vi "FormMain.vi"() -> ()   [LabVIEW 2013]
uses:
  resultShow.vi
panel:
  in  "FormProductsTable":bool
  in  "B030管理":bool
  out "rigStatus 2":string="提示信息"
  in  "判定设定 2":string[][](table)
  in  "参数设定 2":string[][](table)
  out "takesTime":string
  out "表格控件":string[][](table)
  out "FFT范围 2":string[][](table)
  out "输出扭矩":dbl caption="数值 24" format="%.1f Nm"
  in  "打开按钮":bool
  out "rigStatus":string="提示信息"
  out "connectionMode":string
  out "productsName":string
  out "userStatus":string
  out "userName":string
  # "电机/控制器专配专机"
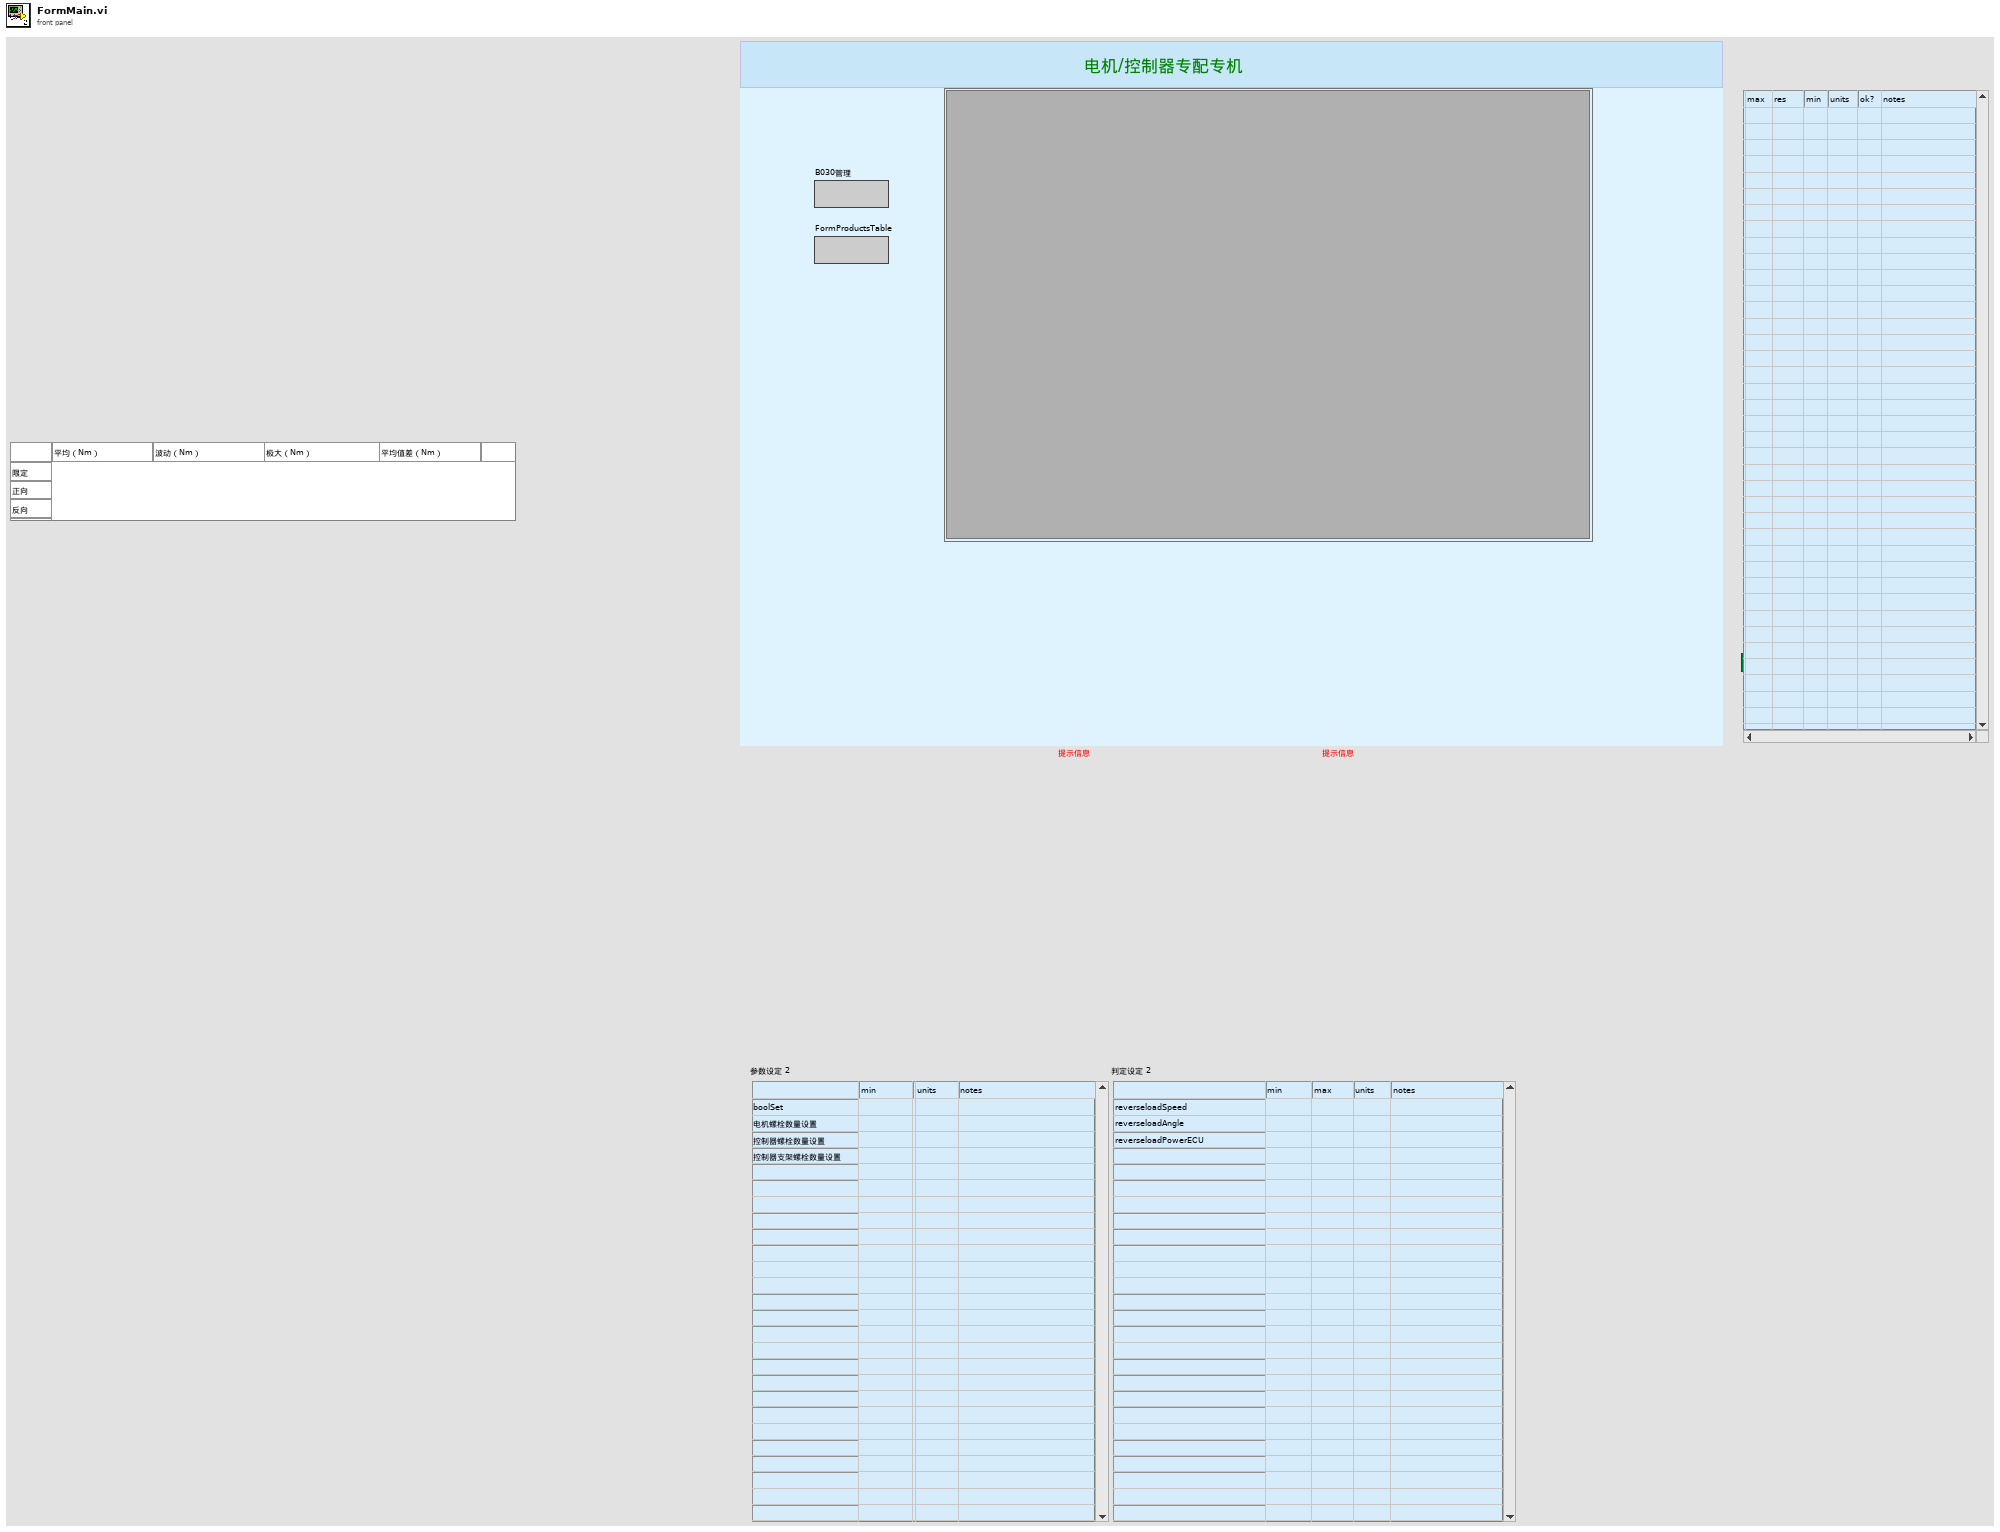
[diagram p1: front panel]
types:
  T1 = enum32{"Invalid", "Standard", "Closed", "Hidden", "Minimized", "Maximized"}
  T2 = cluster{"userCode":string, "userName":string, "userStatus":string, "connectionMode":string, "takesTime":string, "countDone":string, "countOK":string, "countNG":string, "rigStatus":string, "productsName":string, "partCode1":string, "partCode2":string, "partCode3":string}
  T3 = enum32{"Bad", "Idle", "Run top level", "Running"}
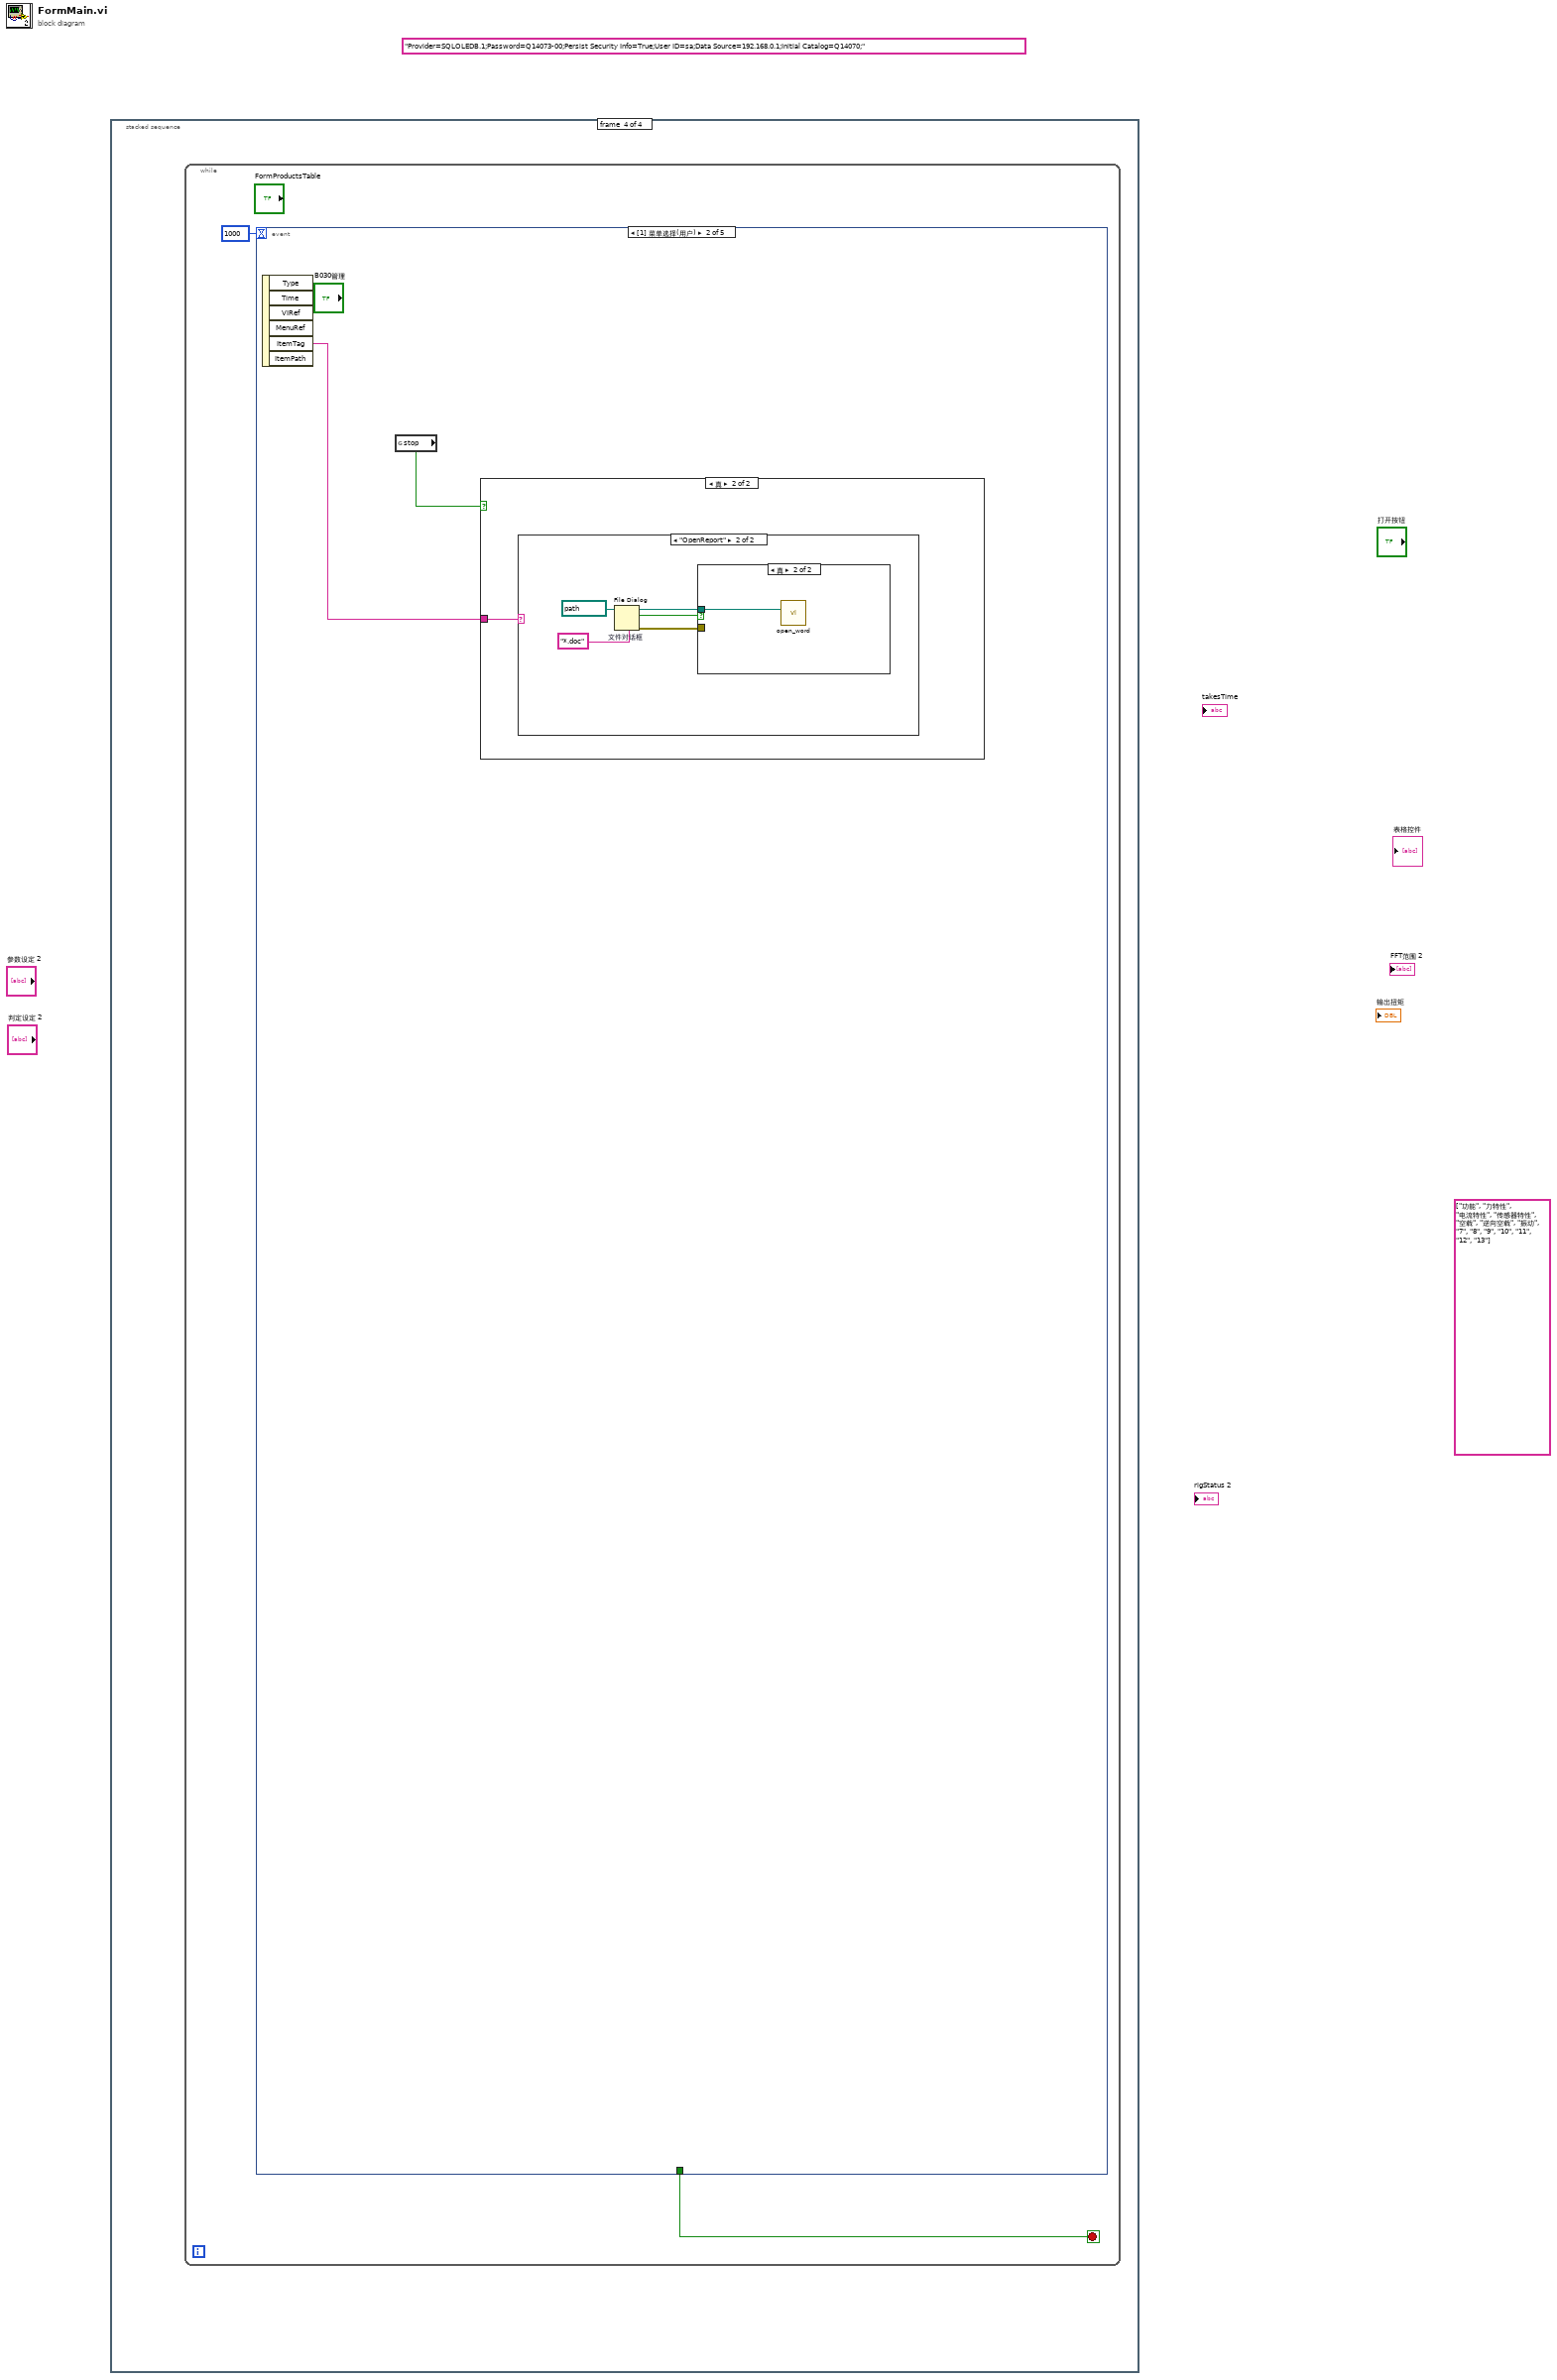
[diagram p0: block diagram]
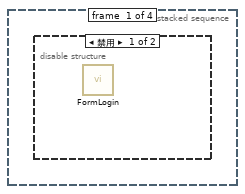
[diagram p2: hidden frame]
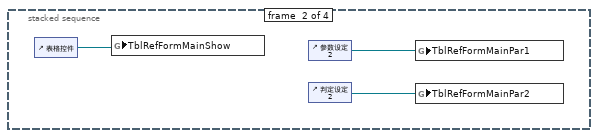
[diagram p4: hidden frame]
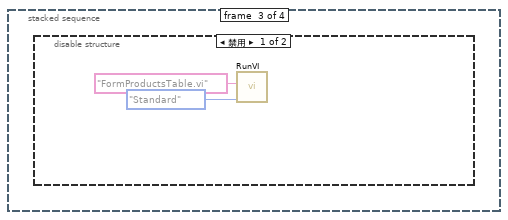
[diagram p5: hidden frame]
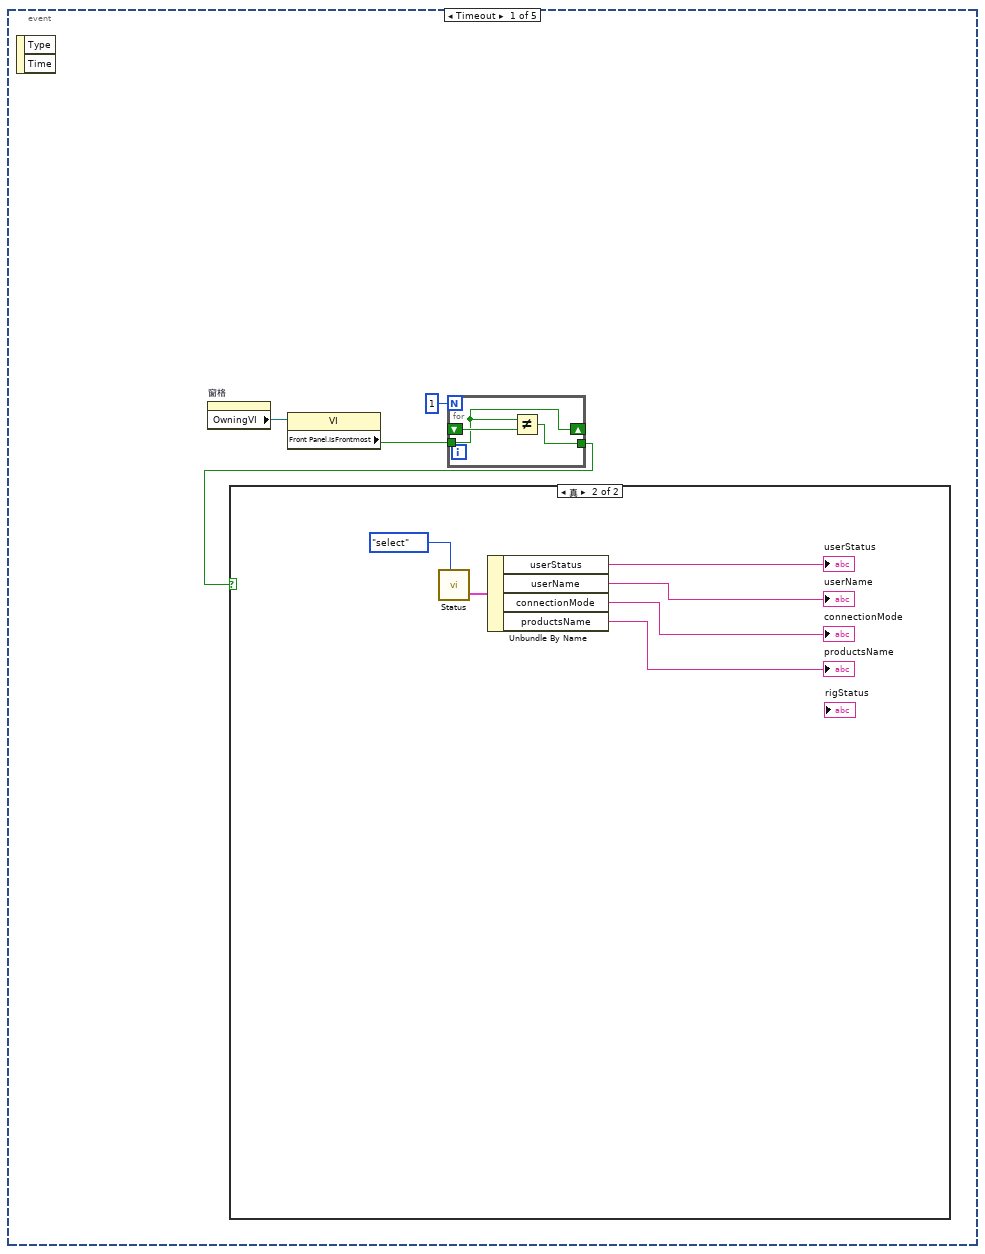
[diagram p7: hidden frame]
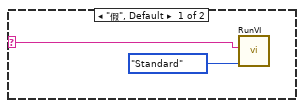
[diagram p10: hidden frame]
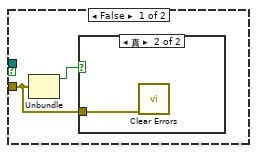
[diagram p11: hidden frame]
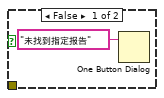
[diagram p12: hidden frame]
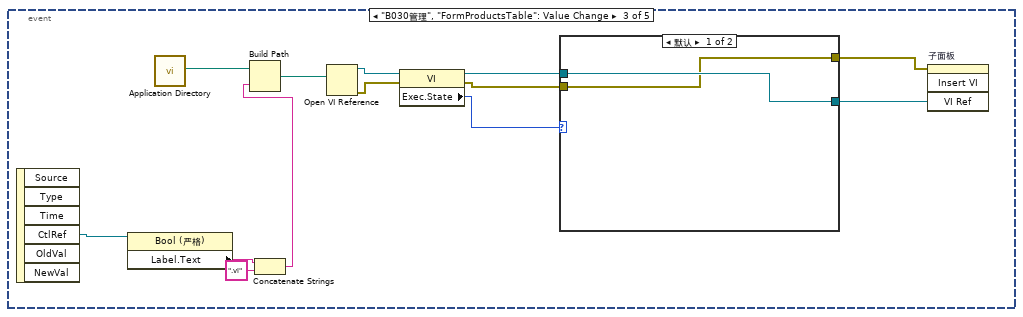
[diagram p13: hidden frame]
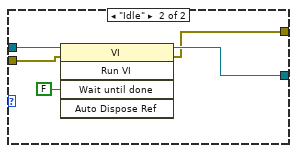
[diagram p14: hidden frame]
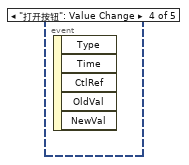
[diagram p15: hidden frame]
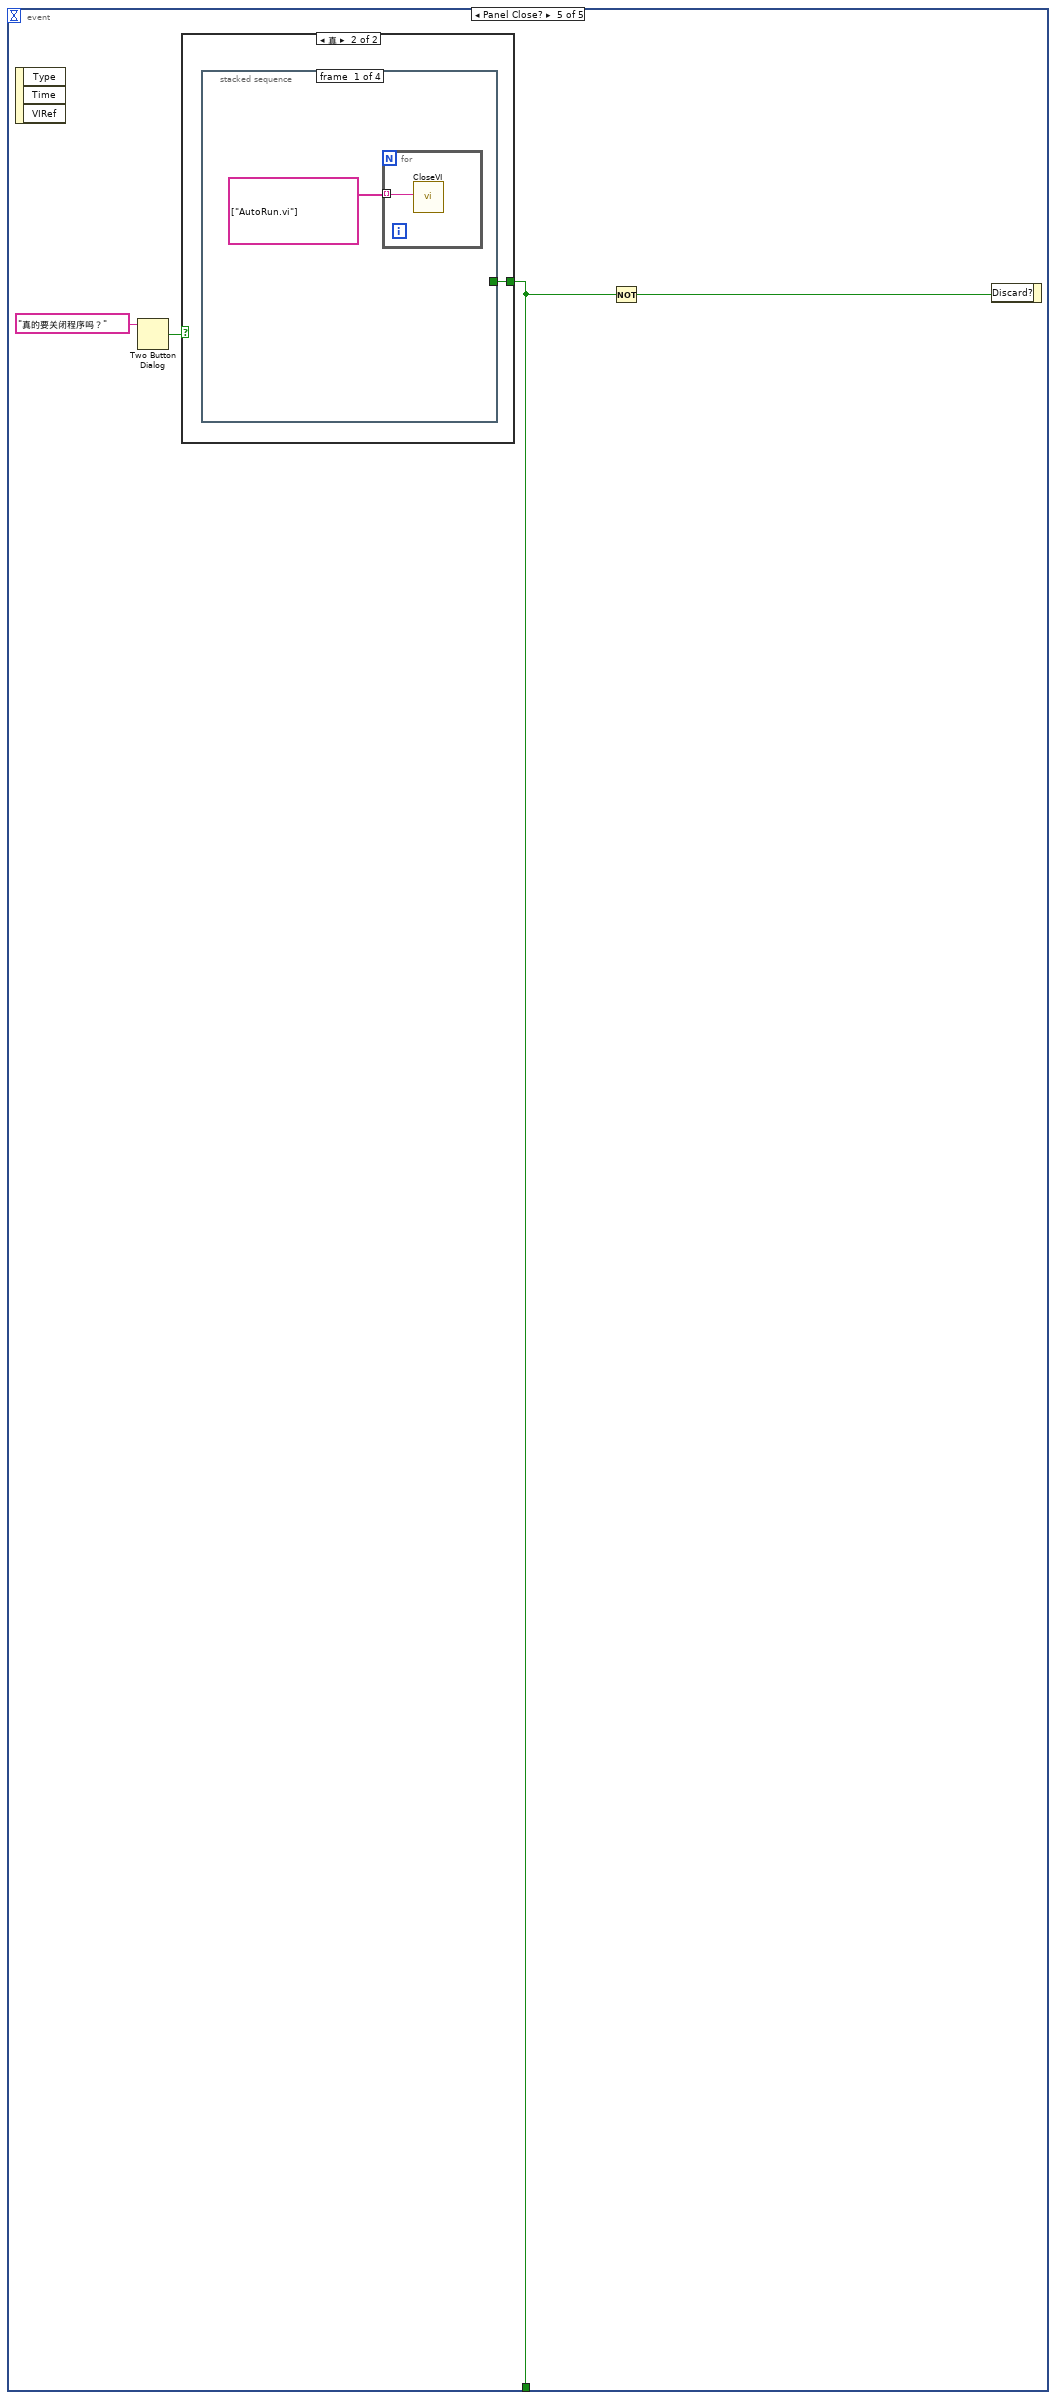
[diagram p16: hidden frame]
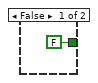
[diagram p17: hidden frame]
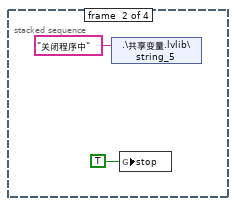
[diagram p18: hidden frame]
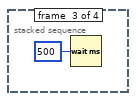
[diagram p19: hidden frame]
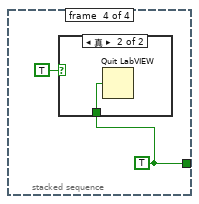
[diagram p20: hidden frame]
diagram:
  (unwired) "Provider=SQLOLEDB.1;Password=Q14073-00;Persist Security Info=True;User ID=sa;Data Source=192.168.0.1;Initial Catalog=Q14070;"
  (unwired) string[] ["功能", "力特性", "电流特性", "传感器特性", "空载", "逆向空载", "振动", "7", "8", "9", "10", "11", "12", "13"] ("字符串[]")
  n1 = stacked-sequence {
    frame #0 {
      n2 = disable-structure shown="禁用" {
        frame Disabled {
          n3 = call "FormLogin.vi"() -> ()  [unwired: 12 in]
        }
        frame Enabled {
        }
      }
    }
    frame #1 {
      n4 = control-ref of="表格控件"() -> (w3:refnum<vi>)
      n5 = global write "resultShow.vi" "TblRefFormMainShow"(w3) -> ()
      n6 = control-ref of="参数设定 2"() -> (w2:refnum<vi>)
      n7 = control-ref of="判定设定 2"() -> (w1:refnum<vi>)
      n8 = global write "resultShow.vi" "TblRefFormMainPar1"(w2) -> ()
      n9 = global write "resultShow.vi" "TblRefFormMainPar2"(w1) -> ()
    }
    frame #2 {
      n10 = disable-structure shown="禁用" {
        frame Disabled {
          n11 = call "RunVI.vi"("状态"=T1."Standard", "名称或相对路径"="FormProductsTable.vi") -> ()  [unwired: 9 in, 1 out]
        }
        frame Enabled {
        }
      }
    }
    frame #3 {
      n12 = while {
        stop <- w7 stop-if-true
        n13 = event shown="[1] 菜单选择(用户)" {
          selector: _ -> [_ _ _ _ _]
          dyn-events: _ -> [_ _ _ _ _]
          timeout: 1000 -> [_ _ _ _ _]
          tunnel: [_ _ _ _ w56] -> w7
          event Timeout {
            n14 = event-data() -> ()  [unwired: 1 in, 2 out]
            n15 = property on="窗格" class="Pane"() -> ("OwningVI"=w11:refnum<vi>)  [unwired: 2 in, 2 out]
            n16 = property class="VI"(reference=w11) -> ("Front Panel.IsFrontmost"=w9:bool)  [unwired: 1 in, 2 out]
            n17 = for {
              N: 1 -> [_]
              shift-right: [w19] -> _
              shift-left: _ -> [w20]
              tunnel: w9 -> [w19]
              tunnel: [w18] -> w8
              n18 = Not Equal?(x=w19, y=w20) -> (x != y?=w18:bool)
            }
            n19 = case shown="真" w8 {
              frame False {
              }
              frame True {
                n20 = call "Status.vi"("模式"=enum16{"select", "insert", "update", "delete"}."select") -> ("元素"=w16:T2)  [unwired: 10 in]
                n21 = Unbundle By Name(w16) -> ("userStatus"=→"userStatus":string, "userName"=→"userName":string, "connectionMode"=→"connectionMode":string, "productsName"=→"productsName":string)
              }
            }
          }
          event Menu Selection (User) {
            n22 = event-data() -> ("ItemTag"=w22:string)  [unwired: 1 in, 5 out]
            n23 = global read "全局 3.vi" "stop"() -> (w21:bool)
            n24 = case shown="真" w21 {
              tunnel: w22 -> [_ w23]
              frame False {
              }
              frame True {
                n25 = case shown="\"OpenReport\"" w23 {
                  selector: w23 -> [w24 _]
                  frame "假", Default {
                    n26 = call "RunVI.vi"("状态"=T1."Standard", "名称或相对路径"=w24) -> ()  [unwired: 9 in, 1 out]
                  }
                  frame "OpenReport" {
                    n27 = File Dialog "文件对话框"(6:"*.doc" ("prompt"), 11:path "D:/报表" ("开始路径")) -> (0:w26:errorcluster, 2:w28:bool, 3:w27:path)  [unwired: 1 in, 5 out]
                    n28 = case shown="真" w28 {
                      tunnel: w27 -> [_ w35]
                      tunnel: w26 -> [w31 _]
                      frame False {
                        n29 = Unbundle(w31) -> ("status"=w32:bool)  [unwired: 2 out]
                        n30 = case shown="真" w32 {
                          tunnel: w31 -> [_ w34]
                          frame False {
                            n31 = One Button Dialog(message="未找到指定报告" ("消息")) -> ()  [unwired: 1 in, 1 out]
                          }
                          frame True {
                            n32 = call <vilib>:"Clear Errors.vi"("error in (no error)"=w34) -> ()  [unwired: 6 in, 1 out]
                          }
                        }
                      }
                      frame True {
                        n33 = call "open_word.vi"("所选路径"=w35) -> ()  [unwired: 11 in]
                      }
                    }
                  }
                }
              }
            }
          }
          event "B030管理", "FormProductsTable": Value Change {
            n34 = event-data() -> ("CtlRef"=w48:refnum<vi>)  [unwired: 1 in, 5 out]
            n35 = property class="Bool (严格)"(reference=w48) -> ("Label.Text"=w38:string)  [unwired: 1 in, 2 out]
            n36 = call <vilib>:"Application Directory.vi"() -> ("Application Directory"=w47:path)
            n37 = Concatenate Strings(w38, ".vi" ("字符串")) -> (w36:string)
            n38 = Build Path(base path=w47, name or relative path=w36) -> (appended path=w46:path)
            n39 = Open VI Reference(vi path=w46) -> (vi reference=w45:refnum<vi>, error out=w44:errorcluster)  [unwired: 5 in]
            n40 = property class="VI"(reference=w45, error in=w44) -> (reference out=w41:refnum<vi>, error out=w40:errorcluster, "Exec.State"=w43:T3)
            n41 = case shown="默认" w43 {
              tunnel: [w50 w52] -> w42
              tunnel: w41 -> [w50 w55]
              tunnel: w40 -> [w49 w54]
              tunnel: [w49 w51] -> w39
              frame Default {
              }
              frame "Idle" {
                n42 = invoke class="VI" method="Run VI"(reference=w55, error in=w54, "Wait until done"=FALSE ("结束前等待")) -> (reference out=w52:refnum<vi>, error out=w51:errorcluster)  [unwired: 2 in, 3 out]
              }
            }
            n43 = invoke on="子面板" class="子面板" method="Insert VI"(error in=w39, "VI Ref"=w42) -> ()  [unwired: 2 in, 4 out]
          }
          event "打开按钮": Value Change {
            n44 = event-data() -> ()  [unwired: 1 in, 5 out]
          }
          event Panel Close? {
            n45 = event-data() -> ()  [unwired: 1 in, 3 out]
            n46 = Two Button Dialog(message="真的要关闭程序吗？" ("消息")) -> (T button?=w57:bool)  [unwired: 2 in]
            n47 = case shown="真" w57 {
              tunnel: [FALSE w61] -> w56
              frame False {
              }
              frame True {
                n48 = stacked-sequence {
                  tunnel: [_ _ _ w68] -> w61
                  frame #0 {
                    n49 = for {
                      tunnel: string[] ["AutoRun.vi"] -> [w63] mode=indexing
                      n50 = call "CloseVI.vi"("名称或相对路径"=w63) -> ()  [unwired: 10 in, 1 out]
                    }
                  }
                  frame #1 {
                    n51 = shared-variable ".\\共享变量.lvlib\\string_5"("关闭程序中" ("string_5")) -> ()  [unwired: 1 in, 1 out]
                    n52 = global write "全局 3.vi" "stop"(TRUE ("布尔 2")) -> ()
                  }
                  frame #2 {
                    n53 = Wait (ms)(milliseconds to wait=u32 500 ("等待时间（毫秒）")) -> ()  [unwired: 1 out]
                  }
                  frame #3 {
                    w68 = TRUE
                    n54 = case shown="真" TRUE {
                      tunnel: w68 -> [_ w69]
                      frame False {
                      }
                      frame True {
                        n55 = Quit LabVIEW(quit? (T)=w69) -> ()
                      }
                    }
                  }
                }
              }
            }
            n56 = Not(x=w56) -> (.not. x?=w58:bool)
            n57 = event-data("Discard?"=w58) -> ()  [unwired: 1 in, 1 out]
          }
        }
      }
    }
  }
